vi "Load Subitems.vi"(7 "defer fp updates?(T)":bool=TRUE, 8 "error in (no error)":errorcluster, 9 "Tag":string, 11 "Application Data in":T1) -> (0 "error out":errorcluster, 1 "item children":string[](array[string]), 3 "Application Data out":T1)   [LabVIEW 2017, in "DSF Simple Explorer.lvlib"]
uses:
  DSF Configuration.llb/DSF Simple Explorer.lvlib
  Application Data.ctl
  Windows/DSF Core.lvlibp/Classes/Configuration/Configuration Session.lvclass
  View Mode.ctl
  Create New Tree Item.vi
  Windows/DSF Core.lvlibp/Classes/Configuration/Read Settings.vi
  Windows/DSF Core.lvlibp/Classes/Configuration/Read Channel.vi
  Windows/DSF Core.lvlibp/Classes/Configuration/Remove ID.vi
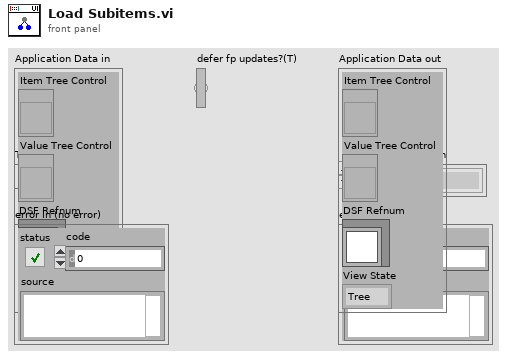
[diagram p1: front panel]
types:
  T1 = typedef "DSF Simple Explorer.lvlib/Application Data.ctl" = cluster{"Item Tree Control":refnum<vi>, "Value Tree Control":refnum<vi>, "DSF Refnum":refnum<class "Configuration Session.lvclass">, "View State":T2}
  T2 = typedef "DSF Simple Explorer.lvlib/View Mode.ctl" = enum16{"Tree", "List"}
  T3 = typedef "DSF Simple Explorer.lvlib/Tree Item Type.ctl" = enum16{"Plugin", "Group", "Transfer", "Channel", "Setting"}
  T4 = typedef "DSF Core.lvlibp/DSF Plugin Info.ctl" = cluster{"components":string[], "timing":T5, "group ids":string[], "settings id":string, "threads":T6[]}
  T5 = typedef "DSF Core.lvlibp/DSF Timing Info.ctl" = cluster{"priority":u64, "decimation":u64, "offset":u64}
  T6 = typedef "DSF Core.lvlibp/DSF Engine Plugin Thread Configuration.ctl" = cluster{"buffer converter settings":T7, "transceiver settings":T7, "custom settings":T7, "processor":i32, "priority offset":i16}
  T7 = typedef "DSF Core.lvlibp/DSF Settings Info.ctl" = cluster{"key":string, "value":string}[]
  T8 = typedef "DSF Simple Explorer.lvlib/Tree Item.ctl" = cluster{"Left Cell String":string, "Child Text":string[], "Child Tag":string, "Glyph Index":i32}
  T9 = typedef "DSF Core.lvlibp/DSF Group Info.ctl" = cluster{"direction":T10, "timing":T5, "transfer ids":string[], "settings id":string, "thread":i32, "timeout behavior":T11}
  T10 = typedef "DSF Core.lvlibp/DSF Direction.ctl" = enum8{"Tx", "Rx"}
  T11 = typedef "DSF Core.lvlibp/DSF Timeout Behavior.ctl" = enum8{"Increment Late Count", "Throw Error"}
  T12 = typedef "DSF Core.lvlibp/DSF Transfer Info.ctl" = cluster{"byte order":T13, "channel ids":string[], "settings id":string}
  T13 = typedef "DSF Core.lvlibp/DSF Byte Order.ctl" = enum8{"big-endian", "little-endian"}
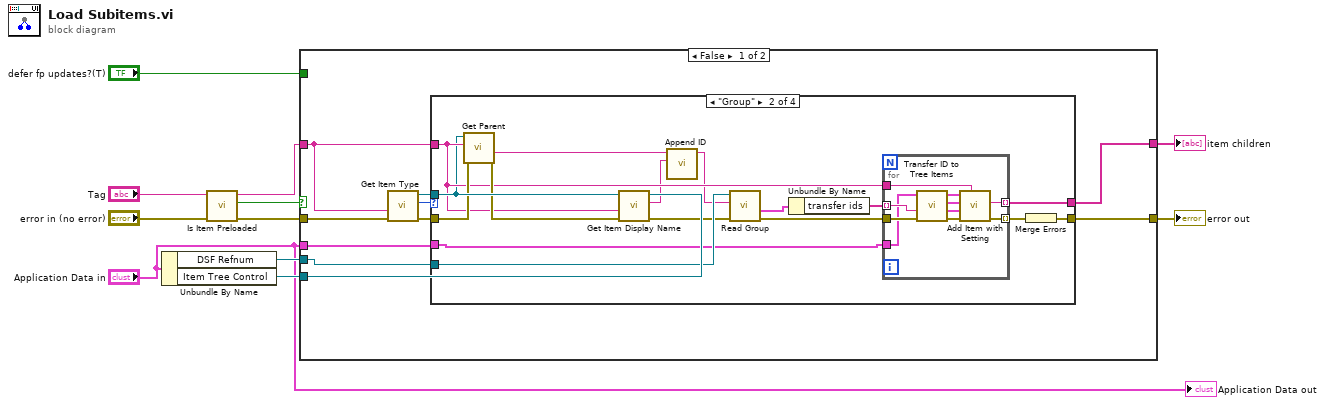
[diagram p0: block diagram]
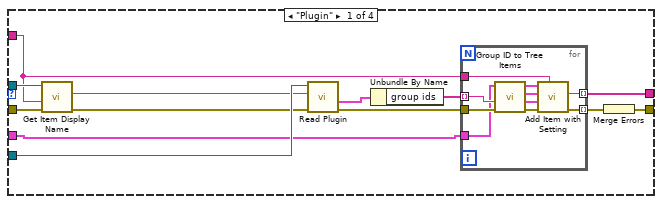
[diagram p2: hidden frame]
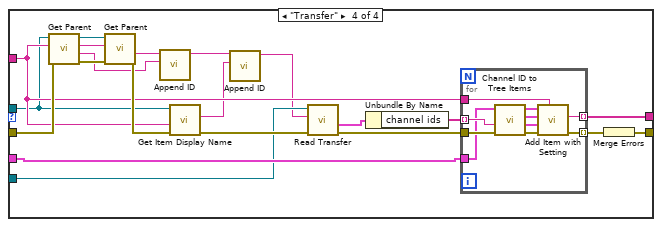
[diagram p4: hidden frame]
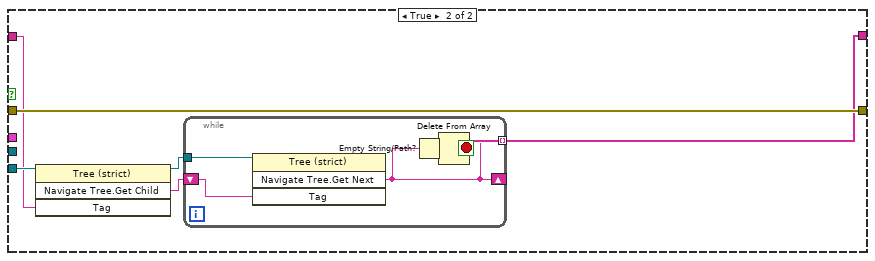
[diagram p5: hidden frame]
diagram:
  n1 = Unbundle By Name("Application Data in") -> ("DSF Refnum"=w4:refnum<class "Configuration Session.lvclass">, "Item Tree Control"=w3:refnum<vi>)
  n2 = call "Is Item Preloaded"("error in (no error)"="error in (no error)", "Tag in"="Tag") -> ("error out"=w8:errorcluster, "replaced"=w10:bool, "Tag out"=w11:string)  [unwired: 7 in]
  n3 = case shown="False" w10 {
    tunnel: w4 -> [w20 _]
    tunnel: w3 -> [w17 w108]
    tunnel: [w18 w109] -> w7
    tunnel: w8 -> [w13 w109]
    tunnel: w11 -> [w12 w107]
    tunnel: [w16 w104] -> w5
    tunnel: "Application Data in" -> [w14 _]
    tunnel: "defer fp updates?(T)" -> [_ _]
    frame False {
      n4 = call "Get Item Type.vi"("error in (no error)"=w13, "Tag"=w12, "TreeControl in"=w17) -> ("error out"=w21:errorcluster, "Item Type"=w19:T3, "TreeControl out"=w15:refnum<vi>)  [unwired: 6 in]
      n5 = case shown="\"Group\"" w19 {
        tunnel: w15 -> [w34 w45 _ w81]
        tunnel: w21 -> [w33 w59 w71 w91]
        tunnel: w20 -> [w32 w58 _ w80]
        tunnel: [w26 w53 w71 w87] -> w18
        tunnel: w12 -> [w23 w49 _ w82]
        tunnel: [w25 w51 _ w84] -> w16
        tunnel: w14 -> [w24 w50 _ w83]
        frame "Plugin" {
          n6 = call "Get Item Display Name.vi"("error in (no error)"=w33, "Tag"=w23, "TreeControl in"=w34) -> ("error out"=w31:errorcluster, "display name"=w22:string)  [unwired: 6 in, 1 out]
          n7 = call "Read Plugin.vi"("error in (no error)"=w31, "Plugin ID"=w22, "Configuration Session in"=w32) -> ("error out"=w28:errorcluster, "value"=w30:T4)  [unwired: 5 in, 2 out]
          n8 = Unbundle By Name(w30) -> ("group ids"=w29:string[])
          n9 = for {
            tunnel: w29 -> [w44] mode=indexing
            tunnel: w28 -> [w43]
            tunnel: [w41] -> w27 mode=indexing
            tunnel: w23 -> [w36]
            tunnel: [w39] -> w25 mode=indexing
            tunnel: w24 -> [w38]
            n10 = call "Group ID to Tree Items.vi"("error in (no error)"=w43, "Group ID"=w44, "Application Data in"=w38) -> ("error out"=w42:errorcluster, "Settings"=w35:T8, "Item"=w40:T8, "Application Data out"=w37:T1)  [unwired: 5 in]
            n11 = call "Add Item with Setting.vi"("Parent Tag"=w36, "error in (no error)"=w42, "Setting"=w35, "Item"=w40, "Application Data in"=w37) -> ("error out"=w41:errorcluster, "new item tag"=w39:string)  [unwired: 4 in, 1 out]
          }
          n12 = Merge Errors(w27) -> (w26:errorcluster)
        }
        frame "Group" {
          n13 = call "Get Parent.vi"("error in (no error)"=w59, "tag"=w49, "TreeControl in"=w45) -> ("error out"=w60:errorcluster, "parent name"=w48:string)  [unwired: 5 in, 2 out]
          n14 = call "Get Item Display Name.vi"("error in (no error)"=w60, "Tag"=w49, "TreeControl in"=w45) -> ("error out"=w57:errorcluster, "display name"=w47:string)  [unwired: 6 in, 1 out]
          n15 = call "Append ID.vi"("name"=w47, "initial id string (\"\")"=w48) -> ("appended id string"=w46:string)  [unwired: 9 in]
          n16 = call "Read Group.vi"("error in (no error)"=w57, "Group ID"=w46, "Configuration Session in"=w58) -> ("error out"=w54:errorcluster, "value"=w56:T9)  [unwired: 5 in, 2 out]
          n17 = Unbundle By Name(w56) -> ("transfer ids"=w55:string[])
          n18 = for {
            tunnel: w55 -> [w70] mode=indexing
            tunnel: w54 -> [w69]
            tunnel: [w67] -> w52 mode=indexing
            tunnel: w49 -> [w63]
            tunnel: [w66] -> w51 mode=indexing
            tunnel: w50 -> [w64]
            n19 = call "Transfer ID to Tree Items.vi"("error in (no error)"=w69, "Transfer ID"=w70, "Application Data in"=w64) -> ("error out"=w68:errorcluster, "Settings"=w61:T8, "Item"=w62:T8, "Application Data out"=w65:T1)  [unwired: 5 in]
            n20 = call "Add Item with Setting.vi"("Parent Tag"=w63, "error in (no error)"=w68, "Setting"=w61, "Item"=w62, "Application Data in"=w65) -> ("error out"=w67:errorcluster, "new item tag"=w66:string)  [unwired: 4 in, 1 out]
          }
          n21 = Merge Errors(w52) -> (w53:errorcluster)
        }
        frame "Channel", "Setting" {
        }
        frame "Transfer" {
          n22 = call "Get Parent.vi"("error in (no error)"=w91, "tag"=w82, "TreeControl in"=w81) -> ("error out"=w76:errorcluster, "parent name"=w75:string, "parent tag"=w79:string, "TreeControl out"=w72:refnum<vi>)  [unwired: 5 in]
          n23 = call "Get Parent.vi"("error in (no error)"=w76, "tag"=w79, "TreeControl in"=w72) -> ("error out"=w92:errorcluster, "parent name"=w78:string)  [unwired: 5 in, 2 out]
          n24 = call "Append ID.vi"("name"=w75, "initial id string (\"\")"=w78) -> ("appended id string"=w77:string)  [unwired: 9 in]
          n25 = call "Get Item Display Name.vi"("error in (no error)"=w92, "Tag"=w82, "TreeControl in"=w81) -> ("error out"=w90:errorcluster, "display name"=w74:string)  [unwired: 6 in, 1 out]
          n26 = call "Append ID.vi"("name"=w74, "initial id string (\"\")"=w77) -> ("appended id string"=w73:string)  [unwired: 9 in]
          n27 = call "Read Transfer.vi"("error in (no error)"=w90, "Transfer ID"=w73, "Configuration Session in"=w80) -> ("error out"=w88:errorcluster, "value"=w89:T12)  [unwired: 5 in, 2 out]
          n28 = Unbundle By Name(w89) -> ("channel ids"=w85:string[])
          n29 = for {
            tunnel: w85 -> [w102] mode=indexing
            tunnel: w88 -> [w101]
            tunnel: [w99] -> w86 mode=indexing
            tunnel: w82 -> [w95]
            tunnel: [w98] -> w84 mode=indexing
            tunnel: w83 -> [w97]
            n30 = call "Channel ID to Tree Items.vi"("error in (no error)"=w101, "Channel ID"=w102, "Application Data in"=w97) -> ("error out"=w100:errorcluster, "Settings"=w94:T8, "Item"=w93:T8, "Application Data out"=w96:T1)  [unwired: 5 in]
            n31 = call "Add Item with Setting.vi"("Parent Tag"=w95, "error in (no error)"=w100, "Setting"=w94, "Item"=w93, "Application Data in"=w96) -> ("error out"=w99:errorcluster, "new item tag"=w98:string)  [unwired: 4 in, 1 out]
          }
          n32 = Merge Errors(w86) -> (w87:errorcluster)
        }
      }
    }
    frame True {
      n33 = invoke class="Tree (strict)" method="Navigate Tree.Get Child"(reference=w108, "Tag"=w107) -> (reference out=w106:refnum<vi>, "Navigate Tree:Get Child"=w103:string)  [unwired: 2 in, 2 out]
      n34 = while {
        tunnel: w106 -> [w113]
        tunnel: [w110] -> w105 mode=indexing
        shift-right: [w110] -> _
        shift-left: w103 -> [w111]
        stop <- w112 stop-if-true
        n35 = invoke class="Tree (strict)" method="Navigate Tree.Get Next"(reference=w113, "Tag"=w111) -> ("Navigate Tree:Get Next Item"=w110:string)  [unwired: 2 in, 3 out]
        n36 = Empty String/Path?(string/path=w110) -> (empty?=w112:bool)
      }
      n37 = Delete From Array(array=w105) -> (array with subset deleted=w104:string[])  [unwired: 2 in, 1 out]
    }
  }
  "error out" <- w7
  "item children" <- w5
  "Application Data out" <- "Application Data in"
